vi "Configure Comparator Mode.vi"(8 "error in (no error)":errorcluster, 10 "Comparator Mode (1: Percent)":u16(ring)=1 items=["Absolute", "Percent", "Sequence"], 11 "VISA resource name":refnum<visa-resource-name>) -> (0 "error out":errorcluster, 3 "VISA resource name out":refnum<visa-resource-name>)   [LabVIEW 2017, in "Agilent E4980.lvlib"]
doc: "Specifies the primary parameter limit values in one of the following three ways:\n\nAbsolute: Tolerance mode based on the absolute parameter values.\nPercent: Tolerance mode based on the deviation percentages.\nSequence: Switches the comparator into sequential mode.\n\n<B>Notes:</B>\n(1) This function clears the primary and secondary parameter limit values."
uses:
  Agilent E4980.lvlib
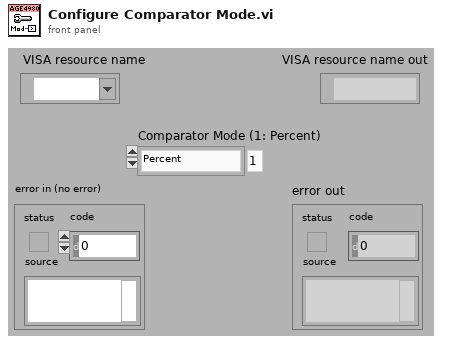
[diagram p1: front panel]
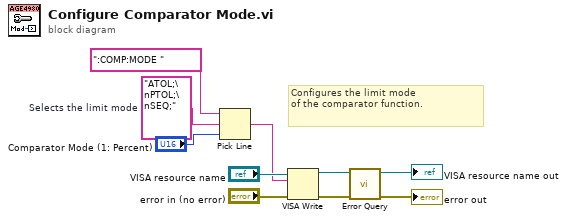
[diagram p0: block diagram]
diagram:
  w9 = "ATOL;\nPTOL;\nSEQ;"  # Selects the limit mode
  # "Configures the limit mode\nof the comparator function."
  n1 = Pick Line(string ("")=":COMP:MODE ", multi-line string=w9, line index="Comparator Mode (1: Percent)") -> (output string=w2:string)
  n2 = VISA Write(VISA resource name="VISA resource name", write buffer=w2, error in (no error)="error in (no error)") -> (VISA resource name out=w6:refnum<visa-resource-name>, error out=w5:errorcluster)  [unwired: 1 out]
  n3 = call "Error Query.vi"("error in (no error)"=w5, "VISA resource name"=w6) -> ("error out"=→"error out":errorcluster, "VISA resource name out"=→"VISA resource name out":refnum<visa-resource-name>)  [unwired: 6 in, 2 out]
